vi "PC TestCode TestFunction.vi"() -> ()   [LabVIEW 2018]
panel:
  in  "Array":u8[](array[numeric])
  out "sum":u8
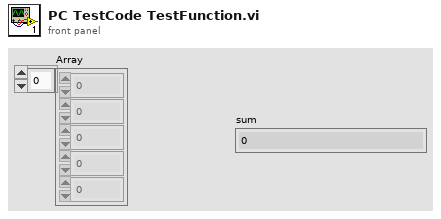
[diagram p1: front panel]
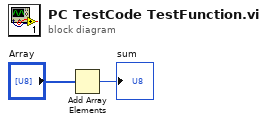
[diagram p0: block diagram]
diagram:
  n1 = Add Array Elements(numeric array="Array") -> (sum=→"sum":u8)
